vi "ClassAppData.Get.vi"(8 "error in (no error)":errorcluster, 9 "Name":string, 10 "Section":string, 11 "Class - App Data in":refnum<class "Class.AppData.lvclass">) -> (0 "error out":errorcluster, 1 "Data Out":variant, 2 "Found":bool, 3 "Class - App Data out":refnum<class "Class.AppData.lvclass">, 4 "String Data":string)   [LabVIEW 2024, in "EQMF.lvlib" / "Config Utils.lvlib" / "Class.AppData.lvclass"]
doc: "<B>AppData Class:</B>\nThe AppData class keeps track of a library of data items that are used by an application. These data items have a name (text string) and value that can be any data type. \n\n<B>AppData.Get VI:</B>\nThis VI is part of the AppData class. This VI will retrieve the AppData item specified by the Data Name input. \n\n<B>Section and Name inputs</B> - The section and name inputs are used to build the data name of the item to be retrieved. If only the Section or only the Name input is populated, then the populated value will be used for the name of the item to retrieve. If both are populated the then the Section and Name will be concatenated with a period separator and that will be used for the name of the item to retrieve.\nEXAMPLE: If Section = \"AA\" and Name = \"BB\" then the name used for the data item will be \"AA.BB\".\n\nData Out - This is a variant containing the value of the item retrieved.\nString Data - This is the string value of the item retrieved. If the item is not a string, then this will be empty. Having this output saves a step of converting a variant to string when the item datatype is a string.\nFound - This is a Boolean output and will be TRUE if the item specified by Data Name existed and was retrieved.\n\n<B>NOTE:</B> If the item specified by Data Name does not exist in the library then this VI will output an empty value with the Found output set to FALSE. No error will be reported."
uses:
  Class.AppData.lvclass
  Class.AppData.lvclass/Class.AppData.ctl
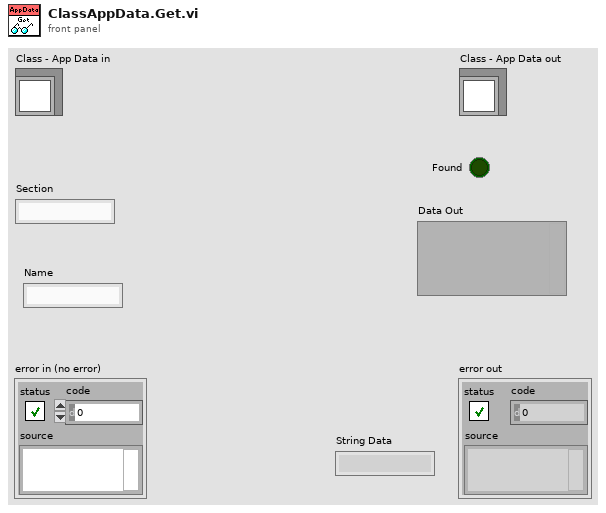
[diagram p1: front panel]
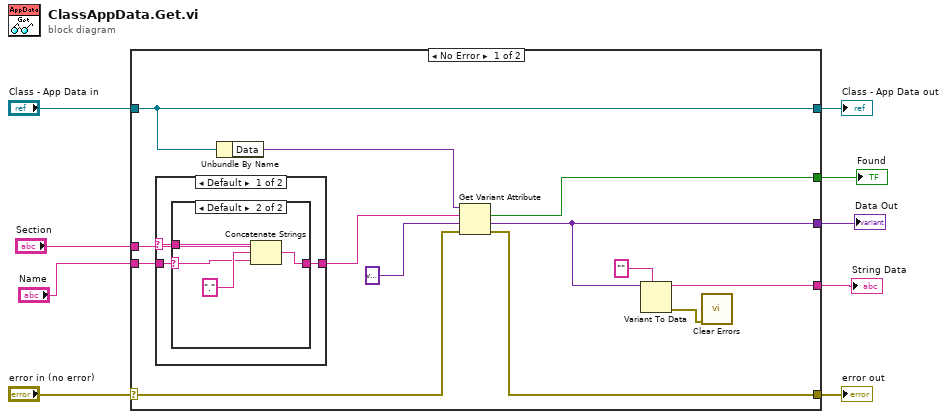
[diagram p0: block diagram]
diagram:
  n1 = case shown="No Error" "error in (no error)" {
    selector: "error in (no error)" -> [w20 w33]
    tunnel: [w18 w33] -> w8
    tunnel: [w22 w32] -> w6
    tunnel: "Class - App Data in" -> [w22 w32]
    tunnel: [w13 _] -> w5
    tunnel: [w17 _] -> w4
    tunnel: "Section" -> [w15 _]
    tunnel: "Name" -> [w14 _]
    tunnel: [w11 _] -> w1
    frame No Error {
      n2 = case shown="Default" w15 {
        selector: w15 -> [w25 _]
        tunnel: w14 -> [w23 w31]
        tunnel: [w24 w31] -> w16
        frame Default {
          n3 = case shown="Default" w23 {
            selector: w23 -> [_ w27]
            tunnel: w25 -> [w26 w30]
            tunnel: [w26 w28] -> w24
            frame "" {
            }
            frame Default {
              n4 = Concatenate Strings(w30, ".", w27) -> (w28:string)
            }
          }
        }
        frame "" {
        }
      }
      n5 = Unbundle By Name(w22) -> ("Data"=w21:variant)
      n6 = Get Variant Attribute(Variant=w21, name=w16, default value (empty Variant)=variant ("value"), error in=w20) -> (found=w17:bool, value=w13:variant, error out=w18:errorcluster)  [unwired: 1 out]
      n7 = Variant To Data(type="", Variant=w13) -> (data=w11:string, error out=w10:errorcluster)  [unwired: 1 in]
      n8 = call <vilib>:"Clear Errors.vi"("error in (no error)"=w10) -> ()  [unwired: 5 in, 2 out]
    }
    frame Error {
    }
  }
  "error out" <- w8
  "Class - App Data out" <- w6
  "Data Out" <- w5
  "Found" <- w4
  "String Data" <- w1
